vi "myRIO_BRig_RT_dataAnalog_valueAI1.vi"() -> (2 "output_valueAI1":i32)   [LabVIEW 2014]
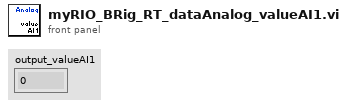
[diagram p1: front panel]
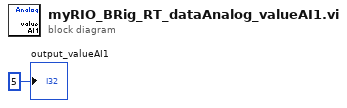
[diagram p0: block diagram]
diagram:
  "output_valueAI1" <- 5 ("output_iBlock")
